vi "checkTimeout.vi"(8 "error in (no error)":errorcluster, 10 "State In":T1, 11 "data passing":T2) -> (0 "error out":errorcluster, 2 "State out":T1, 3 "data passing out":T2)   [LabVIEW 2016]
uses:
  data.ctl
  device/device.ctl
  states.ctl
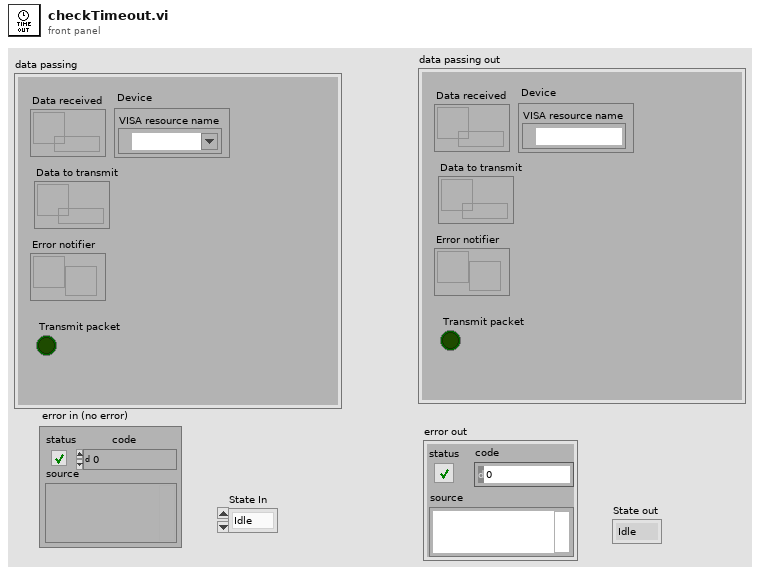
[diagram p1: front panel]
types:
  T1 = typedef "states.ctl" = enum16{"Idle", "Connect", "GetConfig", "Operation", "Disconnect", ""}
  T2 = typedef "data.ctl" = cluster{"Data received":refnum<queue>, "Data to transmit":refnum<queue>, "Error notifier":refnum<notifier>, "Device":T3, "Transmit packet":bool}
  T3 = typedef "device.ctl" = cluster{"VISA resource name":refnum<visa-resource-name>}
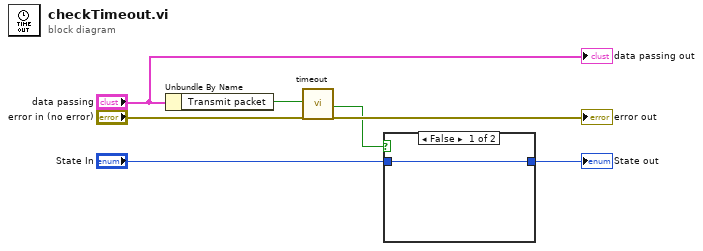
[diagram p0: block diagram]
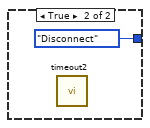
[diagram p2: hidden frame]
diagram:
  n1 = Unbundle By Name("data passing") -> ("Transmit packet"=w7:bool)
  n2 = call "timeout"("Reset"=w7, "error in (no error)"="error in (no error)") -> ("Time has Elapsed"=w4:bool, "error out"=→"error out":errorcluster)  [unwired: 10 in, 6 out]
  n3 = case shown="False" w4 {
    tunnel: "State In" -> [w8 _]
    tunnel: [w8 states."Disconnect" ("Enum")] -> w2
    frame False {
    }
    frame True {
      n4 = call "timeout2"() -> ()  [unwired: 10 in, 2 out]
    }
  }
  "State out" <- w2
  "data passing out" <- "data passing"
